vi "initalize gating(SubVI).vi"(9 "字符串":string, 11 "队列输出":refnum<queue>) -> ()   [LabVIEW 2019, in "SubVI.lvlib"]
uses:
  SubVI.lvlib
  config.ctl
  Instrument.ctl
  lib/QDInstrument.dll
  <vilib>/NI/Modbus Library/API/Master/Modbus Master.lvclass
  lib/Keithley 24XX/Keithley 24XX.lvlib
panel:
  in  "Compliance  Level (0.1)":dbl=0.0001
  in  "2400 resource name":refnum<visa-resource-name>
  # "(真是通道1，假是通道2)"
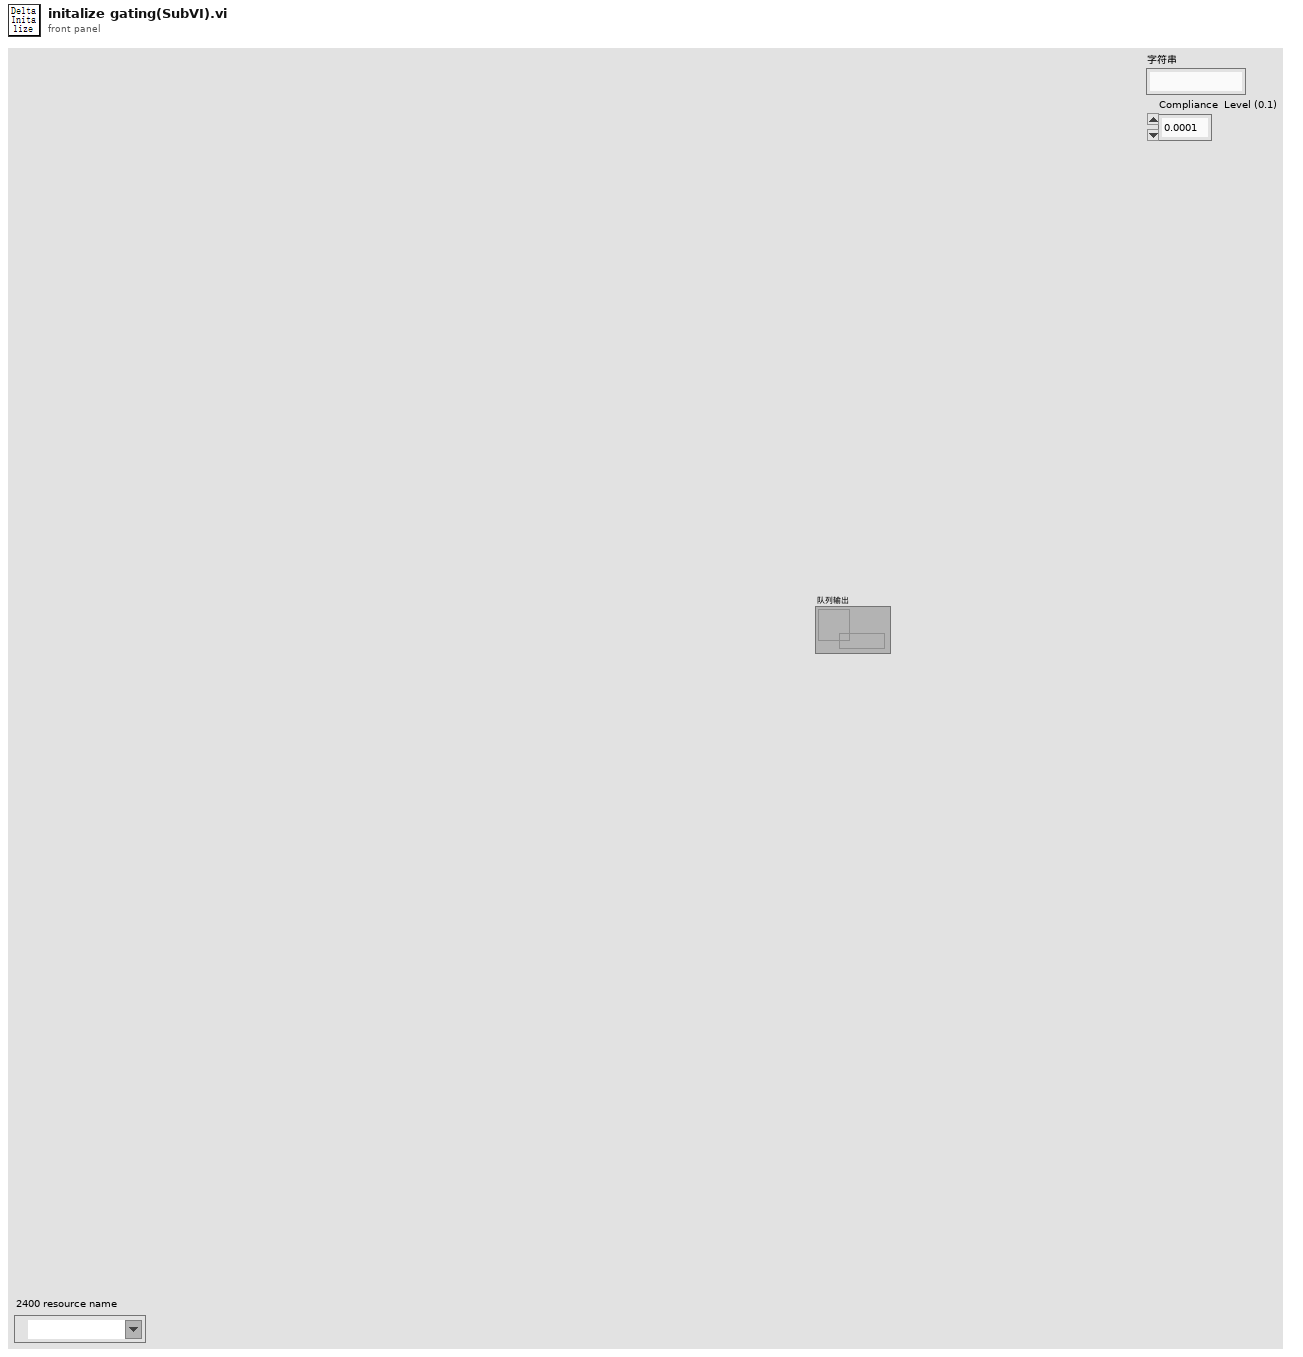
[diagram p1: front panel]
types:
  T1 = cluster{"Baud Rate":u32, "Parity":u16, "Data Bits":u16, "Stop Bits":u16, "Flow Control":u16}
  T2 = typedef "config.ctl" = cluster{"initialize":string, "6221":cluster{"6221 Resource":refnum<visa-resource-name>, "Delta status":bool}, "7001":cluster{"Ch":bool}, "SR830+6221":cluster{"source":u16, "阻抗":dbl, "量程入 4":i32, "量程入 3":i32, "量程入 2":i32, "量程入 1":i32, "电流":dbl, "SR830 2":bool, "SR830 3":bool, "SR830 4":bool, "SR830 1":bool, "VISA 1":refnum<visa-resource-name>, "VISA 2":refnum<visa-resource-name>, "VISA 3":refnum<visa-resource-name>, "VISA 4":refnum<visa-resource-name>, "量程":enum16{"量程每次测量会判定", "量程不变为设定值"}}, "2400":cluster{"2400":bool, "VISA":refnum<visa-resource-name>}, "ch":cluster{"ch str":string, "ch1":bool, "ch2":bool, "布尔":bool}, "error":bool, "数据文件路径":path, "log":cluster{"log路径":path, "log interval":dbl}, "Instrument":T3}
  T3 = typedef "Instrument.ctl" = cluster{"335 Resource":refnum<visa-resource-name>, "Input (0:A)":u16, "Instrument Type":i32, "quantum design":refnum<k24>, "Heater Output (1:1)":u16, "335state":refnum<vi>, "semaphore":T4, "TCP master instance":refnum<class "Modbus Master.lvclass">}
  T4 = typedef "Semaphore RefNum" = refnum<k1>
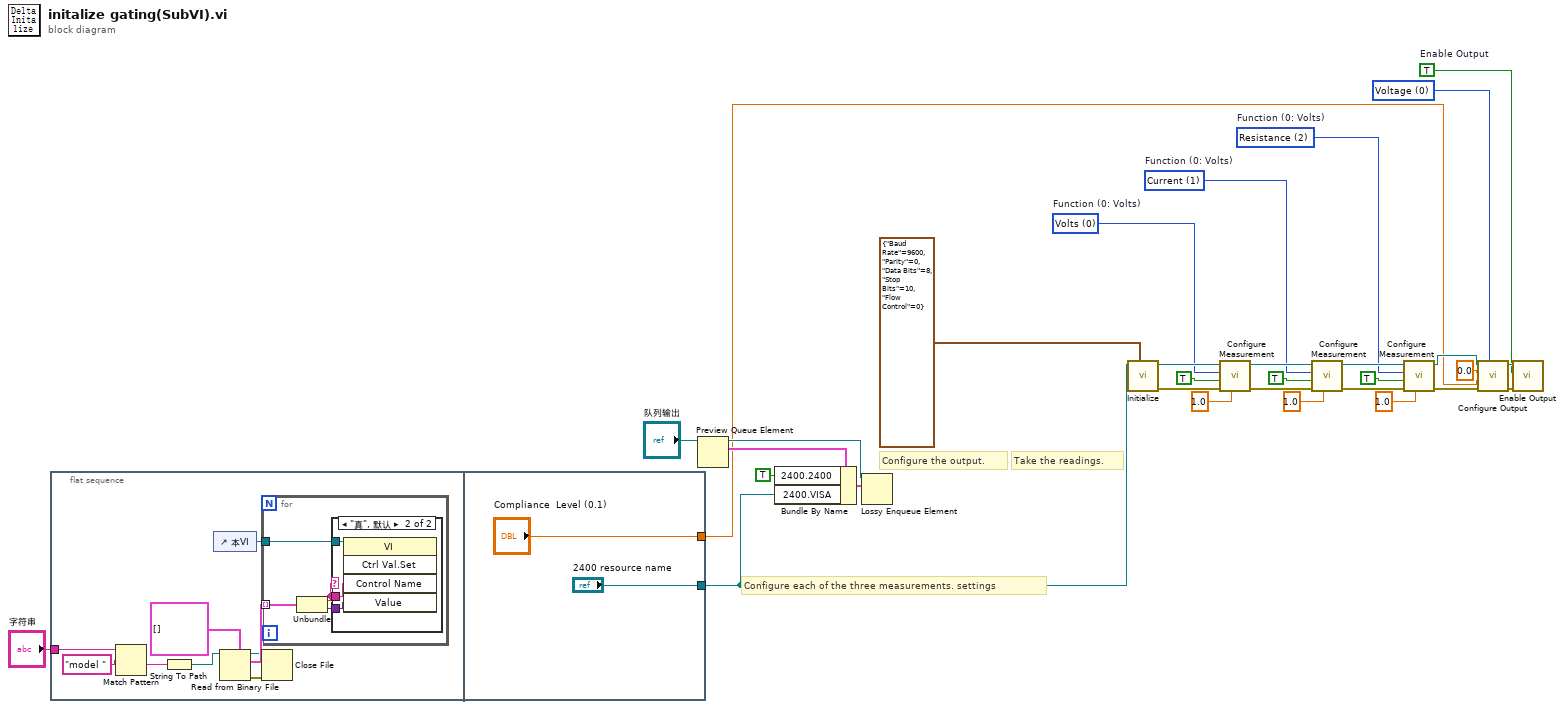
[diagram p0: block diagram]
diagram:
  w4 = u16 0 items=["Voltage", "Current"] ("Source Mode  (0: Voltage)")
  w7 = TRUE  # Enable Output
  w17 = u16 2 items=["Volts", "Current", "Resistance"]  # Function (0: Volts)
  w18 = u16 1 items=["Volts", "Current", "Resistance"]  # Function (0: Volts)
  w19 = u16 0 items=["Volts", "Current", "Resistance"]  # Function (0: Volts)
  # "Take the readings."
  # "Configure the output."
  # "Configure each of the three measurements. settings"
  n1 = flat-sequence {
    tunnel: "字符串" -> [w40]
    tunnel: ["Compliance  Level (0.1)"] -> w3
    tunnel: ["2400 resource name"] -> w2
    frame #0 {
      n2 = Match Pattern(string=w40, regular expression="model " ("正则表达式")) -> (after substring=w39:string)  [unwired: 1 in, 3 out]
      n3 = String To Path(string=w39) -> (path=w36:path)
      n4 = control-ref of="本VI"() -> (w37:refnum<vi>)
      n5 = Read from Binary File(5:cluster{"Name":string, "Variant Data":variant}[] [] ("控件值:获取全部"), 11:w36) -> (0:w32:errorcluster, 2:w34:cluster{"Name":string, "Variant Data":variant}[], 3:w33:refnum<file>)  [unwired: 4 in, 1 out]
      n6 = for {
        tunnel: w34 -> [w44] mode=indexing
        tunnel: w37 -> [w43]
        n7 = Unbundle(w44) -> ("Name"=w41:string, "Variant Data"=w42:variant)
        n8 = case shown="\"真\", 默认" w41 {
          tunnel: w43 -> [_ w47]
          tunnel: w41 -> [_ w46]
          tunnel: w42 -> [_ w45]
          frame "cancel", "load", "model", "ok" {
          }
          frame "真", Default {
            n9 = invoke class="VI" method="Ctrl Val.Set"(reference=w47, "Control Name"=w46, "Value"=w45) -> ()  [unwired: 2 in, 5 out]
          }
        }
      }
      n10 = Close File(refnum=w33, error in=w32) -> ()  [unwired: 2 out]
    }
    frame #1 {
    }
  }
  n11 = Preview Queue Element(queue="队列输出") -> (queue out=w28:refnum<queue>, element=w29:T2)  [unwired: 2 in, 2 out]
  n12 = Bundle By Name(cluster=w29, "2400.2400"=TRUE, "2400.VISA"=w2) -> (w27:T2)
  n13 = Lossy Enqueue Element(queue=w28, element=w27) -> ()  [unwired: 1 in, 4 out]
  n14 = call "Initialize.vi"("Serial Configuration"=T1 {"Baud Rate"=9600, "Parity"=0, "Data Bits"=8, "Stop Bits"=10, "Flow Control"=0}, "VISA resource name"=w2) -> ("error out"=w24:errorcluster, "VISA resource name out"=w25:refnum<visa-resource-name>)  [unwired: 8 in]
  n15 = call "Configure Measurement.vi"("Manual Range (1.0)"=1.0 ("Voltage Manual Range (1.0)"), "error in (no error)"=w24, "Enable Auto Range (T:Enable)"=TRUE ("Enable Voltage Auto Range (T:Enable)"), "Function (0: Volts)"=w19, "VISA resource name"=w25) -> ("error out"=w22:errorcluster, "VISA resource name out"=w23:refnum<visa-resource-name>)  [unwired: 5 in]
  n16 = call "Configure Measurement.vi"("Manual Range (1.0)"=1.0 ("Current Manual Range (1.0)"), "error in (no error)"=w22, "Enable Auto Range (T:Enable)"=TRUE ("Enable Current Auto Range (T:Enable)"), "Function (0: Volts)"=w18, "VISA resource name"=w23) -> ("error out"=w21:errorcluster, "VISA resource name out"=w20:refnum<visa-resource-name>)  [unwired: 5 in]
  n17 = call "Configure Measurement.vi"("Manual Range (1.0)"=1.0 ("Resistance Manual Range (1.0)"), "error in (no error)"=w21, "Enable Auto Range (T:Enable)"=TRUE ("Enable Resistance Auto Range (T:Enable)"), "Function (0: Volts)"=w17, "VISA resource name"=w20) -> ("error out"=w6:errorcluster, "VISA resource name out"=w5:refnum<visa-resource-name>)  [unwired: 5 in]
  n18 = call "Configure Output.vi"("Source Mode  (0: Voltage)"=w4, "error in (no error)"=w6, "Compliance  Level (0.1)"=w3, "Output Level (0)"=0.0, "VISA resource name"=w5) -> ("error out"=w8:errorcluster, "VISA resource name out"=w9:refnum<visa-resource-name>)  [unwired: 5 in]
  n19 = call "Enable Output.vi"("error in (no error)"=w8, "Enable Output (T: Enable)"=w7, "VISA resource name"=w9) -> ()  [unwired: 7 in, 2 out]
